vi "setForceSetpointToForceMeasured.vi"(8 "error in (no error)":errorcluster, 11 "Model in":refnum<class "Model.lvclass">) -> (0 "error out":errorcluster, 3 "Model out":refnum<class "Model.lvclass">)   [LabVIEW 2015]
uses:
  <userlib>/Common/Devices/ForceSensorCalculator/ForceSensorCalculator/ForceSensorCalculator.lvclass
  ApplicationElements/SystemController/SystemController.lvclass
  Model.lvclass
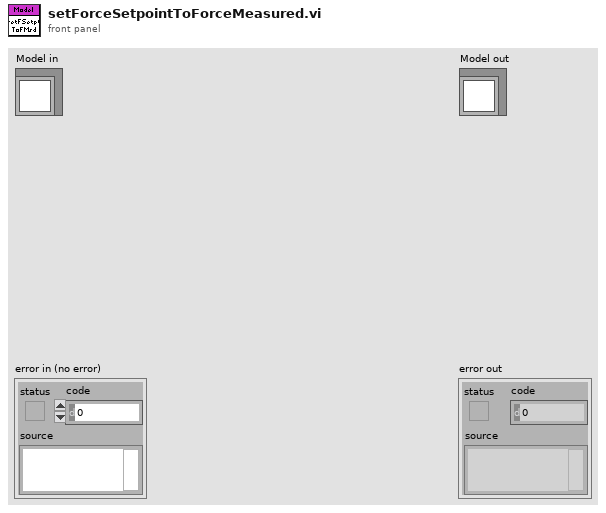
[diagram p1: front panel]
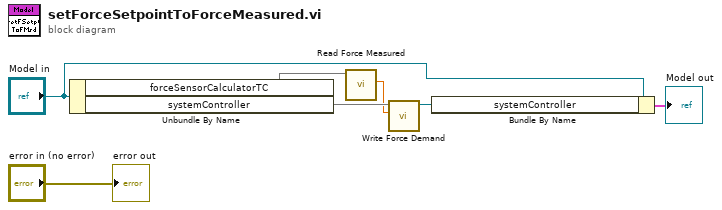
[diagram p0: block diagram]
diagram:
  n1 = Unbundle By Name("Model in") -> ("forceSensorCalculatorTC"=w4, "systemController"=w3)
  n2 = call <userlib>:"Read Force Measured.vi"("ForceSensor in"=w4) -> ("Force Demand"=w2:dbl[unit])  [unwired: 9 in, 1 out]
  n3 = call "Write Force Demand.vi"("Force Demand"=w2, "SystemController in"=w3) -> ("SystemController out"=w1:refnum<class "SystemController.lvclass">)  [unwired: 9 in]
  n4 = Bundle By Name(cluster="Model in", "systemController"=w1) -> (→"Model out":cluster{})
  "error out" <- "error in (no error)"
